vi "test4.vi"   [LabVIEW 2012]
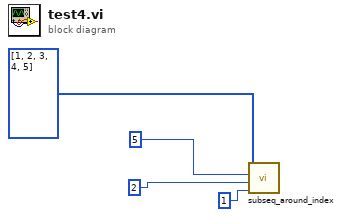
[diagram p0: block diagram]
diagram:
  n1 = call "subseq_around_index.vi"("length around index 2"=1 ("array length 2"), "index 2"=2 ("array length 2"), "array length 2"=5, "Array 3"=i16[] [1, 2, 3, 4, 5]) -> ()  [unwired: 7 in, 1 out]
